vi "S2C_VLFT10_Proc_DateAndTime.vi"(8 "Error In":errorcluster, 11 "Time":string) -> (0 "Error Out":errorcluster, 3 "Result":string)   [LabVIEW 2015]
uses:
  Fornax/VIs/PolyDriver/Typedefs/TimeCommand.ctl
  Fornax/VIs/PolyDriver/S2C_FORNAX_Poly_TimeCommand.vi
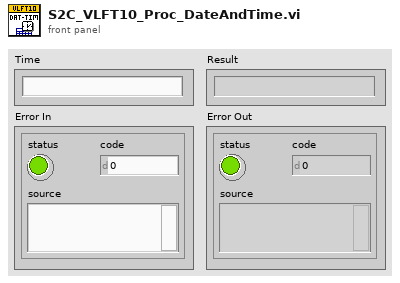
[diagram p1: front panel]
types:
  T1 = typedef "TimeCommand.ctl" = i16
  T2 = cluster{"Driver":string, "Command":string, "Return":string, "Parameters":string, "Timeout":dbl}
  T3 = cluster{"Partition":string, "Message":string, "M_Command":T1, "M_Value":string}
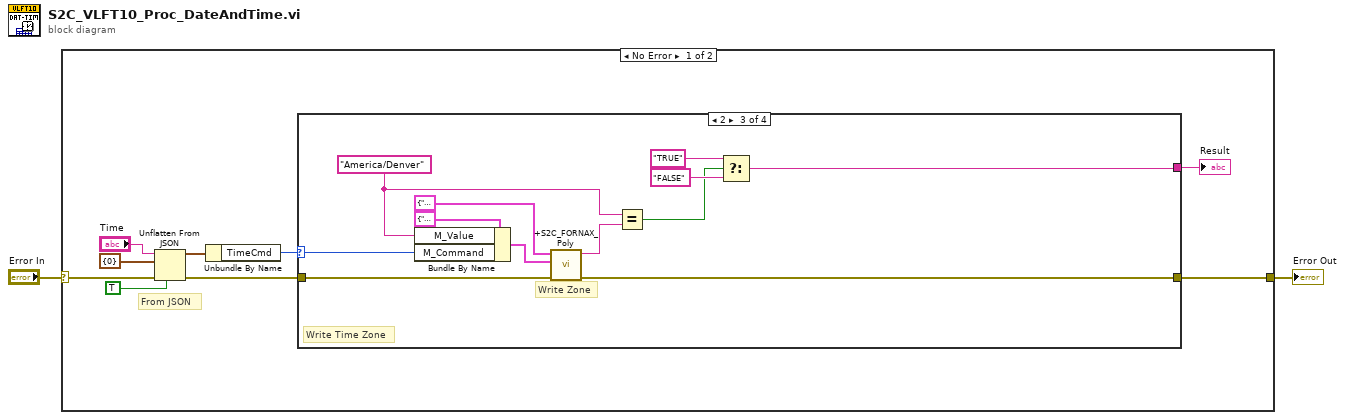
[diagram p0: block diagram]
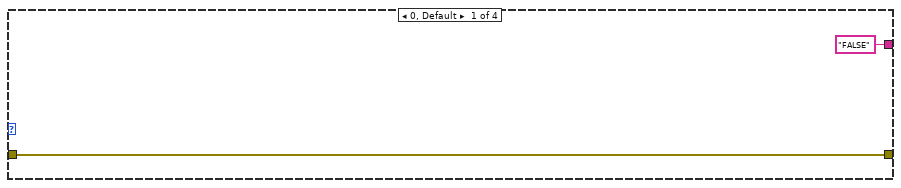
[diagram p2: hidden frame]
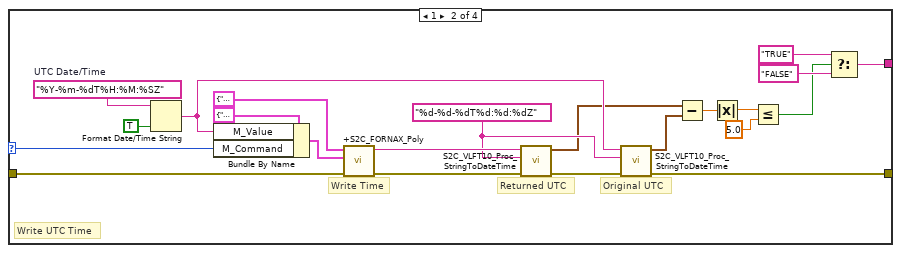
[diagram p3: hidden frame]
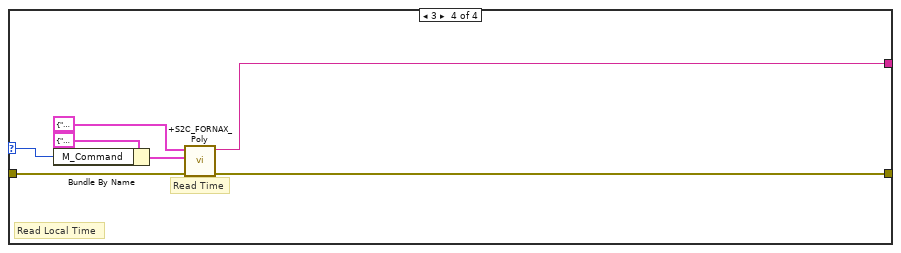
[diagram p4: hidden frame]
diagram:
  n1 = case shown="No Error" "Error In" {
    selector: "Error In" -> [w4 w55]
    tunnel: [w8 w55] -> w1
    frame No Error {
      # "From JSON"
      n2 = Unflatten From JSON(JSON string="Time", type and defaults=cluster{"TimeCmd":T1} {"TimeCmd"=0}, default null elements? (F)=TRUE, error in (no error)=w4) -> (value=w9:cluster{"TimeCmd":T1}, error out=w11:errorcluster)  [unwired: 3 in]
      n3 = Unbundle By Name(w9) -> ("TimeCmd"=w5:T1)
      n4 = case shown="2" w5 {
        selector: w5 -> [_ w33 w45 w52]
        tunnel: w11 -> [w13 w35 w47 w54]
        tunnel: [w13 w19 w39 w51] -> w8
        tunnel: ["FALSE" ("Response") w16 w41 w50] -> w7
        frame 0, Default {
        }
        frame 1 {
          w25 = "%d-%d-%dT%d:%d:%dZ" ("format string")
          w31 = "%Y-%m-%dT%H:%M:%SZ"  # UTC Date/Time
          # "Write UTC Time"
          # "Original UTC"
          # "Returned UTC"
          # "Write Time"
          n5 = Format Date/Time String(time format string (%c)=w31, UTC format=TRUE) -> (date/time string=w26:string)  [unwired: 1 in]
          n6 = Bundle By Name(cluster=T3 {"Partition"="Default", "Message"="TimeCommand", "M_Command"=0, "M_Value"=""} ("TimeCommand"), "M_Value"=w26, "M_Command"=w33) -> (w34:T3)
          n7 = call-poly "+S2C_FORNAX_Poly.vi"("Error In"=w35, "TimeCommand"=w34, "Settings"=T2 {"Driver"="Fornax", "Command"="TimeCommand", "Return"="M_UtcTime", "Parameters"="", "Timeout"=10.0}) -> ("Error Out"=w29:errorcluster, "Response"=w28:string)  [unwired: 7 in]
          n8 = call "S2C_VLFT10_Proc_StringToDateTime.vi"("Error In"=w29, "Format String"=w25, "DateTime String"=w28) -> ("Error Out"=w27:errorcluster, "TimeStamp"=w24:timestamp)  [unwired: 7 in]
          n9 = call "S2C_VLFT10_Proc_StringToDateTime.vi"("Error In"=w27, "Format String"=w25, "DateTime String"=w26) -> ("Error Out"=w19:errorcluster, "TimeStamp"=w23:timestamp)  [unwired: 7 in]
          n10 = Subtract(x=w24, y=w23) -> (x-y=w22:dbl)
          n11 = Absolute Value(x=w22) -> (abs(x)=w21:dbl)
          n12 = Less Or Equal?(x=w21, y=5.0) -> (x <= y?=w15:bool)
          n13 = Select(t="TRUE", s=w15, f="FALSE") -> (s? t:f=w16:string)
        }
        frame 2 {
          w37 = "America/Denver"
          # "Write Time Zone"
          # "Write Zone"
          n14 = Bundle By Name(cluster=T3 {"Partition"="Default", "Message"="TimeCommand", "M_Command"=0, "M_Value"=""} ("TimeCommand"), "M_Value"=w37, "M_Command"=w45) -> (w46:T3)
          n15 = call-poly "+S2C_FORNAX_Poly.vi"("Error In"=w47, "TimeCommand"=w46, "Settings"=T2 {"Driver"="Fornax", "Command"="TimeCommand", "Return"="M_TimeZone", "Parameters"="", "Timeout"=10.0}) -> ("Error Out"=w39:errorcluster, "Response"=w38:string)  [unwired: 7 in]
          n16 = Equal?(x=w37, y=w38) -> (x = y?=w36:bool)
          n17 = Select(t="TRUE", s=w36, f="FALSE") -> (s? t:f=w41:string)
        }
        frame 3 {
          # "Read Local Time"
          # "Read Time"
          n18 = Bundle By Name(cluster=T3 {"Partition"="Default", "Message"="TimeCommand", "M_Command"=0, "M_Value"=""} ("TimeCommand"), "M_Command"=w52) -> (w53:T3)
          n19 = call-poly "+S2C_FORNAX_Poly.vi"("Error In"=w54, "TimeCommand"=w53, "Settings"=T2 {"Driver"="Fornax", "Command"="TimeCommand", "Return"="M_LocalTime", "Parameters"="", "Timeout"=10.0}) -> ("Error Out"=w51:errorcluster, "Response"=w50:string)  [unwired: 7 in]
        }
      }
      "Result" <- w7
    }
    frame Error {
    }
  }
  "Error Out" <- w1
